vi "Init PWM.vi"(5 "Phase-Correct (F)":bool, 7 "GPIO":i32, 8 "error in (no error)":errorcluster, 10 "Enable (F)":bool, 11 "VISA resource name in":refnum<visa-resource-name>) -> (0 "error out":errorcluster, 3 "VISA resource name":refnum<visa-resource-name>)   [LabVIEW 2024, in "CTIPicoVISA.lvlib"]
uses:
  CTIPicoVISA.lvlib
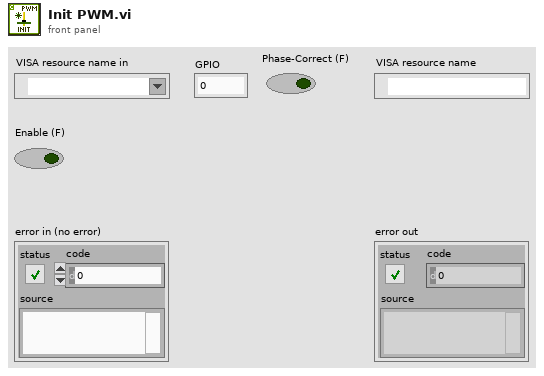
[diagram p1: front panel]
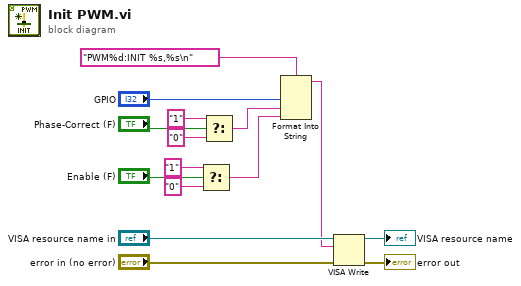
[diagram p0: block diagram]
diagram:
  n1 = Select(t="1", s="Enable (F)", f="0") -> (s? t:f=w1:string)
  n2 = Select(t="1", s="Phase-Correct (F)", f="0") -> (s? t:f=w2:string)
  n3 = Format Into String(format string="PWM%d:INIT %s,%s\n", "GPIO", w2, w1) -> (resulting string=w9:string)  [unwired: 2 in, 1 out]
  n4 = VISA Write(VISA resource name="VISA resource name in", write buffer=w9, error in (no error)="error in (no error)") -> (VISA resource name out=→"VISA resource name":refnum<visa-resource-name>, error out=→"error out":errorcluster)  [unwired: 1 out]
